vi "change tablevalu.vi"(9 "Active Cell":T1, 10 "Value":dbl, 11 "Item Names":string[][](array[string])) -> (2 "tablevalue out":string[][](array[string]))   [LabVIEW 2011]
uses:
  <vilib>/Utility/miscctls.llb/LVRowAndColumnTypeDef.ctl
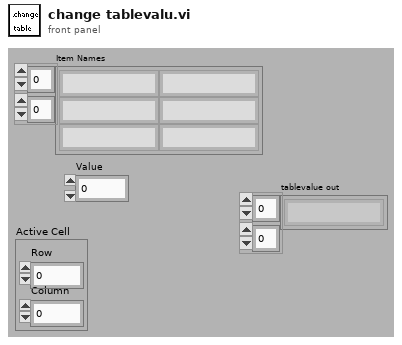
[diagram p1: front panel]
types:
  T1 = typedef "LVRowAndColumnTypeDef.ctl" = cluster{"Row":i32, "Column":i32}
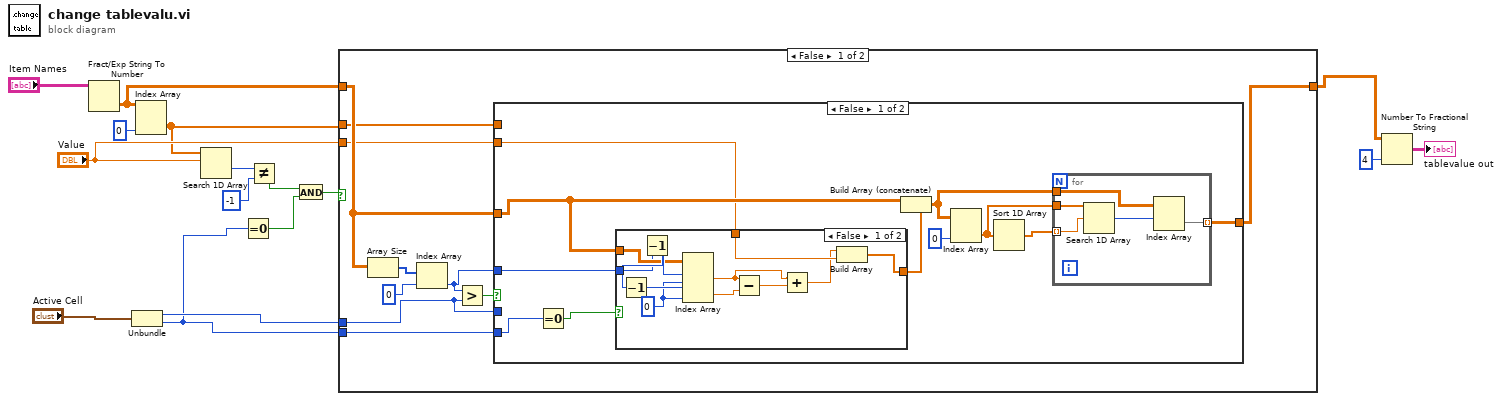
[diagram p0: block diagram]
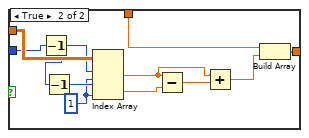
[diagram p2: hidden frame]
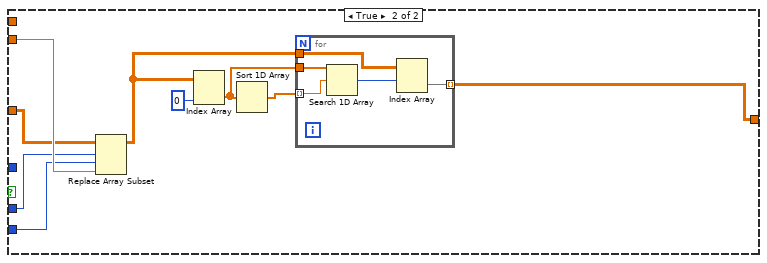
[diagram p3: hidden frame]
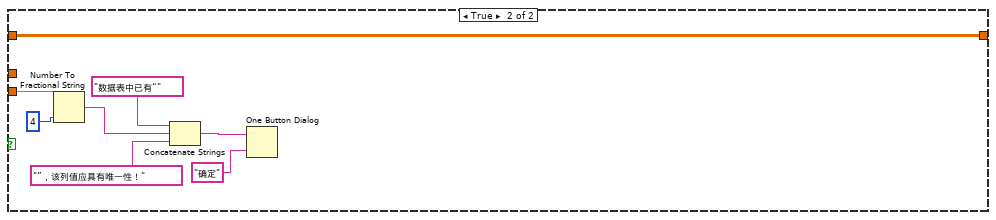
[diagram p4: hidden frame]
diagram:
  n1 = Fract/Exp String To Number(string="Item Names") -> (number=w8:dbl[][])  [unwired: 4 out]
  n2 = Unbundle("Active Cell") -> ("Row"=w6:i32, "Column"=w5:i32)
  n3 = Index Array(array=w8, index (col)=0 ("disabled index (col)")) -> (element=w9:dbl[])  [unwired: 1 in]
  n4 = Search 1D Array(1D array=w9, element="Value") -> (index of element=w15:i32)  [unwired: 1 out]
  n5 = Equal To 0?(x=w5) -> (x = 0?=w11:bool)
  n6 = Not Equal?(x=w15, y=-1) -> (x != y?=w12:bool)
  n7 = And(x=w12, y=w11) -> (x .and. y?=w10:bool)
  n8 = case shown="False" w10 {
    tunnel: "Value" -> [w22 w85]
    tunnel: w9 -> [w20 _]
    tunnel: w8 -> [w24 w79]
    tunnel: w6 -> [w23 _]
    tunnel: w5 -> [w21 _]
    tunnel: [w17 w79] -> w3
    frame False {
      n9 = Array Size(array=w24) -> (size(s)=w19:i32[])
      n10 = Index Array(array=w19, index=0) -> (element=w18:i32)
      n11 = Greater?(x=w18, y=w23) -> (0:w25:bool)
      n12 = case shown="False" w25 {
        tunnel: w24 -> [w35 w67]
        tunnel: w23 -> [_ w71]
        tunnel: w22 -> [w33 w73]
        tunnel: w21 -> [w37 w72]
        tunnel: w20 -> [_ _]
        tunnel: w18 -> [w34 _]
        tunnel: [w27 w65] -> w17
        frame False {
          n13 = Equal To 0?(x=w37) -> (x = 0?=w36:bool)
          n14 = case shown="False" w36 {
            tunnel: w35 -> [w46 w64]
            tunnel: w34 -> [w45 w63]
            tunnel: w33 -> [w44 w56]
            tunnel: [w47 w54] -> w32
            frame False {
              w51 = 0
              n15 = Decrement(x=w45) -> (x-1=w52:i32)
              n16 = Decrement(x=w52) -> (x-1=w53:i32)
              n17 = Index Array(array=w46, index (row) #1=w52, index (col) #1=w51, index (row) #2=w53, index (col) #2=w51) -> (element #1=w49:dbl, element #2=w50:dbl)
              n18 = Subtract(x=w49, y=w50) -> (x-y=w48:dbl)
              n19 = Add(x=w49, y=w48) -> (x+y=w43:dbl)
              n20 = Build Array(w43, w44) -> (w47:dbl[])
            }
            frame True {
              w60 = 1
              n21 = Decrement(x=w63) -> (x-1=w61:i32)
              n22 = Decrement(x=w61) -> (x-1=w62:i32)
              n23 = Index Array(array=w64, index (row) #1=w61, index (col) #1=w60, index (row) #2=w62, index (col) #2=w60) -> (element #1=w58:dbl, element #2=w59:dbl)
              n24 = Subtract(x=w58, y=w59) -> (x-y=w57:dbl)
              n25 = Add(x=w58, y=w57) -> (x+y=w55:dbl)
              n26 = Build Array(w56, w55) -> (w54:dbl[])
            }
          }
          n27 = Build Array (concatenate)(w35, w32) -> (w28:dbl[][])
          n28 = Index Array(array=w28, index (col)=0 ("disabled index (col)")) -> (element=w29:dbl[])  [unwired: 1 in]
          n29 = Sort 1D Array(array=w29) -> (sorted array=w30:dbl[])
          n30 = for {
            tunnel: w30 -> [w41] mode=indexing
            tunnel: w29 -> [w42]
            tunnel: w28 -> [w40]
            tunnel: [w38] -> w27 mode=indexing
            n31 = Search 1D Array(1D array=w42, element=w41) -> (index of element=w39:i32)  [unwired: 1 out]
            n32 = Index Array(array=w40, index (row)=w39) -> (element=w38:dbl[])  [unwired: 1 in]
          }
        }
        frame True {
          n33 = Replace Array Subset(array=w67, new element=w73, index (row)=w71, index (col)=w72) -> (w66:dbl[][])
          n34 = Index Array(array=w66, index (col)=0 ("disabled index (col)")) -> (element=w68:dbl[])  [unwired: 1 in]
          n35 = Sort 1D Array(array=w68) -> (sorted array=w69:dbl[])
          n36 = for {
            tunnel: w69 -> [w77] mode=indexing
            tunnel: w68 -> [w78]
            tunnel: w66 -> [w76]
            tunnel: [w74] -> w65 mode=indexing
            n37 = Search 1D Array(1D array=w78, element=w77) -> (index of element=w75:i32)  [unwired: 1 out]
            n38 = Index Array(array=w76, index (row)=w75) -> (element=w74:dbl[])  [unwired: 1 in]
          }
        }
      }
    }
    frame True {
      n39 = Number To Fractional String(number=w85, precision (6)=i16 4) -> (F-format string=w82:string)  [unwired: 1 in, 1 out]
      n40 = Concatenate Strings("数据表中已有“", w82, "”，该列值应具有唯一性！" ("string")) -> (w80:string)
      n41 = One Button Dialog(message=w80, button name ("OK")="确定") -> ()  [unwired: 1 out]
    }
  }
  n42 = Number To Fractional String(number=w3, precision (6)=i16 4) -> (F-format string=→"tablevalue out":string[][])  [unwired: 2 out]
